vi "Row Col  Range Format.vi"(1 "Column":i32 caption="列", 2 "Row":i32 caption="行") -> (0 "Output String":string caption="输出字符串")   [LabVIEW 2017]
doc: "将行数和列数转换为Excel格式A1、A2...和B1、B2....等。"
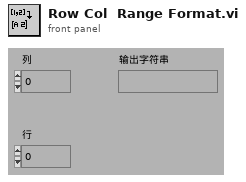
[diagram p1: front panel]
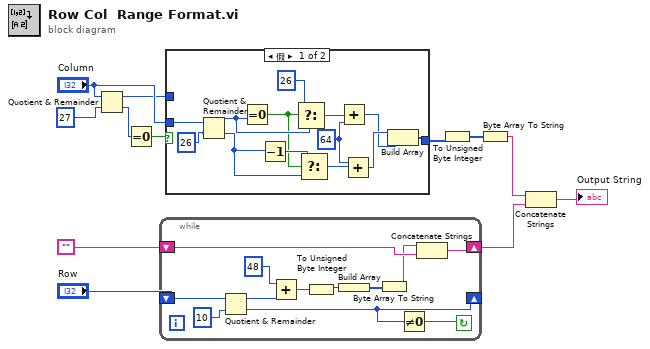
[diagram p0: block diagram]
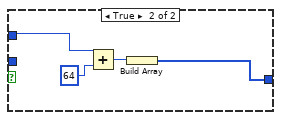
[diagram p2: hidden frame]
diagram:
  n1 = Quotient & Remainder(x="Column", y=27) -> (x-y*floor(x/y)=w8:i32, floor(x/y)=w9:i32)
  n2 = Equal To 0?(x=w9) -> (x = 0?=w10:bool)
  n3 = while {
    shift-left: "Row" -> [w24]
    shift-right: [w15] -> _
    shift-left: "" -> [w14]
    shift-right: [w17] -> w2
    stop <- w16 continue-if-true
    n4 = Quotient & Remainder(x=w24, y=10) -> (x-y*floor(x/y)=w22:i32, floor(x/y)=w15:i32)
    n5 = Add(x=48, y=w22) -> (x+y=w20:i32)
    n6 = To Unsigned Byte Integer(number=w20) -> (unsigned 8bit integer=w19:u8)
    n7 = Build Array(w19) -> (w18:u8[])
    n8 = Byte Array To String(unsigned byte array=w18) -> (string=w13:string)
    n9 = Not Equal To 0?(x=w15) -> (x != 0?=w16:bool)
    n10 = Concatenate Strings(w13, w14) -> (w17:string)
  }
  n11 = case shown="假" w10 {
    tunnel: "Column" -> [w37 _]
    tunnel: w8 -> [_ w41]
    tunnel: [w26 w40] -> w7
    frame False {
      w25 = 64
      n12 = Quotient & Remainder(x=w37, y=26) -> (x-y*floor(x/y)=w34:i32, floor(x/y)=w31:i32)
      n13 = Equal To 0?(x=w34) -> (x = 0?=w32:bool)
      n14 = Decrement(x=w31) -> (x-1=w33:i32)
      n15 = Select(t=26, s=w32, f=w34) -> (s? t:f=w30:i32)
      n16 = Select(t=w33, s=w32, f=w31) -> (s? t:f=w29:i32)
      n17 = Add(x=w30, y=w25) -> (x+y=w27:i32)
      n18 = Add(x=w25, y=w29) -> (x+y=w28:i32)
      n19 = Build Array(w28, w27) -> (w26:i32[])
    }
    frame True {
      n20 = Add(x=w41, y=64) -> (x+y=w38:i32)
      n21 = Build Array(w38) -> (w40:i32[])
    }
  }
  n22 = To Unsigned Byte Integer(number=w7) -> (unsigned 8bit integer=w6:u8[])
  n23 = Byte Array To String(unsigned byte array=w6) -> (string=w3:string)
  n24 = Concatenate Strings(w3, w2) -> (→"Output String":string)
